vi "test.vi"() -> ()   [LabVIEW 2020, in "EPA 1065.lvlib" / "Gas Analyzer Drift 1065-550.lvlib"]
uses:
  Gas Analyzer Drift 1065-550.lvlib
panel:
  in  "Registerkartenelement":T1(tab)
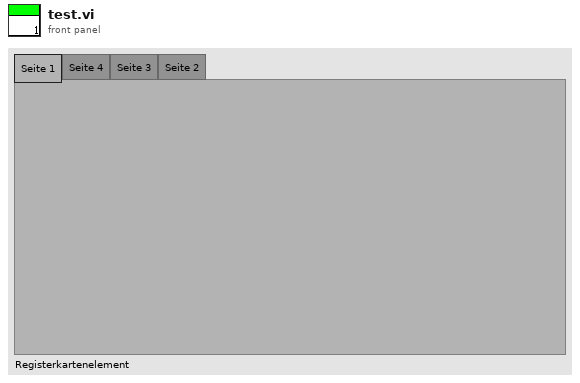
[diagram p1: front panel]
types:
  T1 = enum32{"Seite 1", "Seite 4", "Seite 3", "Seite 2"}
  T2 = enum32{"Page Enabled", "Page Disabled", "Page Disabled & Grayed"}
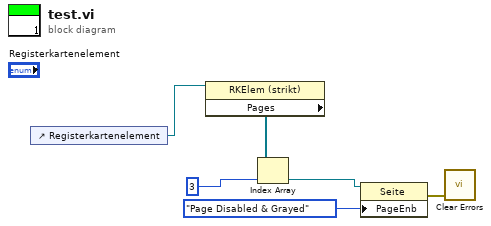
[diagram p0: block diagram]
diagram:
  n1 = control-ref of="Registerkartenelement"() -> (w2:refnum<vi>)
  n2 = property class="RKElem (strikt)"(reference=w2) -> ("Pages"=w1:refnum<vi>[])  [unwired: 1 in, 2 out]
  n3 = Index Array(array=w1, index=3 ("Index")) -> (element=w4:refnum<vi>)
  n4 = property class="Seite"(reference=w4, "PageEnb"=T2."Page Disabled & Grayed" ("Aktiv-Status der Seite")) -> (error out=w3:errorcluster)  [unwired: 1 in, 1 out]
  n5 = call <vilib>:"Clear Errors.vi"("error in (no error)"=w3) -> ()  [unwired: 5 in, 2 out]
